vi "Get Counter Configuration.vi"(8 "error in":errorcluster, 11 "Parent Ref":T1=18446744073709551615 format="%.0x") -> (0 "error out":errorcluster, 2 "Max Count":dbl, 3 "Parent Ref Out":T1=18446744073709551615 format="%.0x")   [LabVIEW 2015, in "Protection and Rolling Counter Addon System Explorer.lvlib"]
uses:
  Protection and Rolling Counter Addon System Explorer.lvlib
  <vilib>/NI Veristand/Custom Device API/Custom Device Item Ref.ctl
  Shared/SubVIs/GUID Lookup.vi
  <vilib>/NI Veristand/Custom Device API/Get Item Property (Variant).vi
  Shared/Protection and Rolling Counter Addon Shared.lvlib
  <vilib>/NI VeriStand/Custom Device API/Custom Device API.lvlib
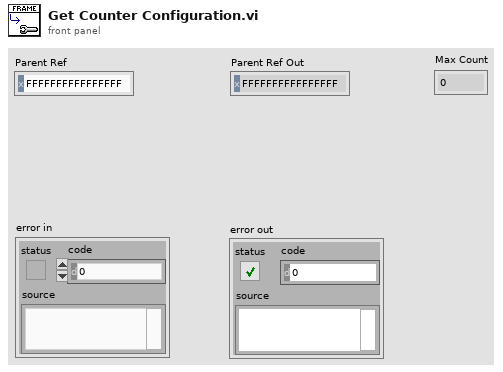
[diagram p1: front panel]
types:
  T1 = typedef "Custom Device API.lvlib/Custom Device Item Ref.ctl" = u64
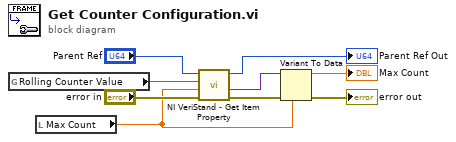
[diagram p0: block diagram]
diagram:
  n1 = global read "GUID Lookup.vi" "Rolling Counter Value"() -> (w1:string)
  n2 = local read "Max Count"() -> (w2:dbl)
  n3 = call-poly <vilib>:"NI VeriStand - Get Item Property.vi"("error in (no error)"="error in", "Default Value"=w2, "Property Name"=w1, "Item Ref in"="Parent Ref") -> ("error out"=w8:errorcluster, "Value"=w4:variant, "Item Ref out"=→"Parent Ref Out":T1)  [unwired: 4 in, 1 out]
  n4 = Variant To Data(error in=w8, type=w2, Variant=w4) -> (data=→"Max Count":dbl, error out=→"error out":errorcluster)
